vi "Example Threshold - PressureReached Callback.vi"(4 "PressureReached":refnum<user-event>, 5 "Event Data":cluster{"sender":refnum<k24>, "pressure":i32}, 6 "Control Ref":refnum<k24>, 7 "Event Common Data":T1) -> ()   [LabVIEW 2010]
uses:
  C:/tf/play/labview/Tinkerforge.dll
  Tinkerforge.dll
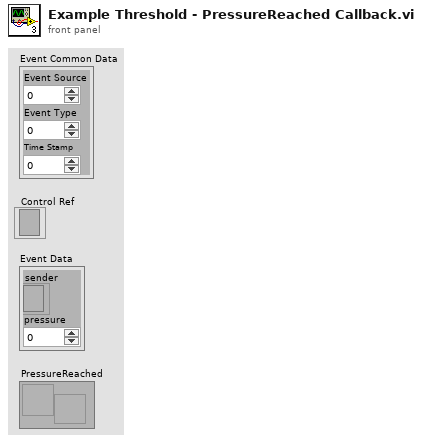
[diagram p1: front panel]
types:
  T1 = cluster{"Event Source":i32, "Event Type":u32, "Time Stamp":u32}
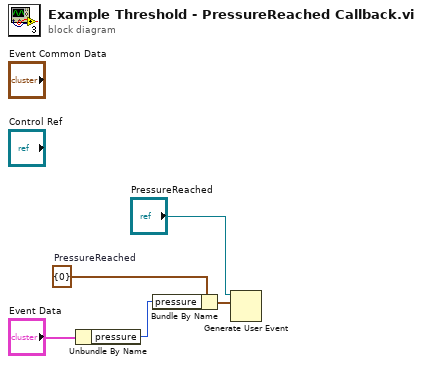
[diagram p0: block diagram]
diagram:
  w3 = cluster{"pressure":i32} {"pressure"=0}  # PressureReached
  n1 = Unbundle By Name("Event Data") -> ("pressure"=w1:i32)
  n2 = Bundle By Name(cluster=w3, "pressure"=w1) -> (w4:cluster{"pressure":i32})
  n3 = Generate User Event(user event="PressureReached", event data cluster=w4) -> ()  [unwired: 1 in, 2 out]
